vi "FarFiledCamInit.vi"(2 "error in (no error)":errorcluster caption="error in（no error）") -> (0 "error out":errorcluster)   [LabVIEW 2018]
panel:
  out "MinValue":u32
  out "MaxValue":u32
  out "CameraName":string
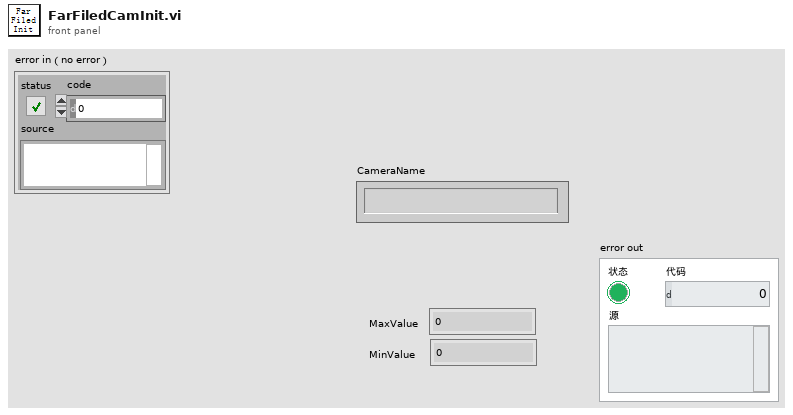
[diagram p1: front panel]
types:
  T1 = typedef "Image Type" = u32
  T2 = typedef "IMAQ Image.ctl" = refnum<image>
  T3 = cluster{"示波器":cluster{"Channel (0:Channel 1)":enum16{"Channel 1", "Channel 2", "Channel 3", "Channel 4"}, "电压范围":dbl, "触发电压":dbl, "时间范围":dbl, " 示波器VISA":refnum<visa-resource-name>, "时间范围 标签":u64, "电压范围 标签":u64, "触发电压 标签":u64, "输入阻抗/Ω":u64}, "光谱仪":cluster{"SpecDataReference":refnum<queue>, "grating center":dbl, "Exposure Time (s)":dbl, "是否进行详细设置":bool, " 开始通信检查":bool, "通信成功？":bool, "波长":dbl}, " 近场相机":cluster{"曝光时间/100us":dbl, "模拟增益":i32, "控制套接字":i32, "IP 地址":string, " 采集套接字":i32, "  版本号":i32, "ImageData":T2, "  增益最大":i32, "  增益最小":i32, " 曝光最大":i32, " 曝光最小":i32, " 帧速":i32, " 同步切换":i32, "  曝光缩放":i32}, " 偏振仪":cluster{"电压范围":u64, "触发电压":u64, "时间范围":u64, "波长范围":enum16{"可见光 400-700nm", "近红外 700-1100nm"}, "可见光偏振测量仪VISA":refnum<visa-resource-name>, "近红外偏振测量仪VISA":refnum<visa-resource-name>}, " 功率计":cluster{"通道":enum16{"Channel 1", "Channel 2"}, "工作波长":u32, "单位":u64, "时间范围":u64, "IP地址":string, "端口":u32}, "能量计":cluster{"通道":enum16{"Channel 1", "Channel 2"}, "工作波长":u32, "单位":u64, "时间范围":u64, "IP地址":string, "端口":u32, "能量计量程":enum16{"200uJ", "20uJ", "2uJ", "200nJ"}}, "电机":cluster{"Channel (0:Channel 1)":enum16{"Channel 1", "Channel 2", "Channel 3", "Channel 4"}, "电压范围":u64, "触发电压":u64, "时间范围":u64}, " 远场相机":cluster{"曝光时间":i32, "模拟增益":i32, "控制套接字":i32, "IP 地址":string, " 采集套接字":i32, "  版本号":i32, "ImageData":T2, "  增益最大":i32, "  增益最小":i32, " 曝光最大":i32, " 曝光最小":i32, " 帧速":i32, " 同步切换":i32, "  曝光缩放":i32, "ImageData B":T2}}
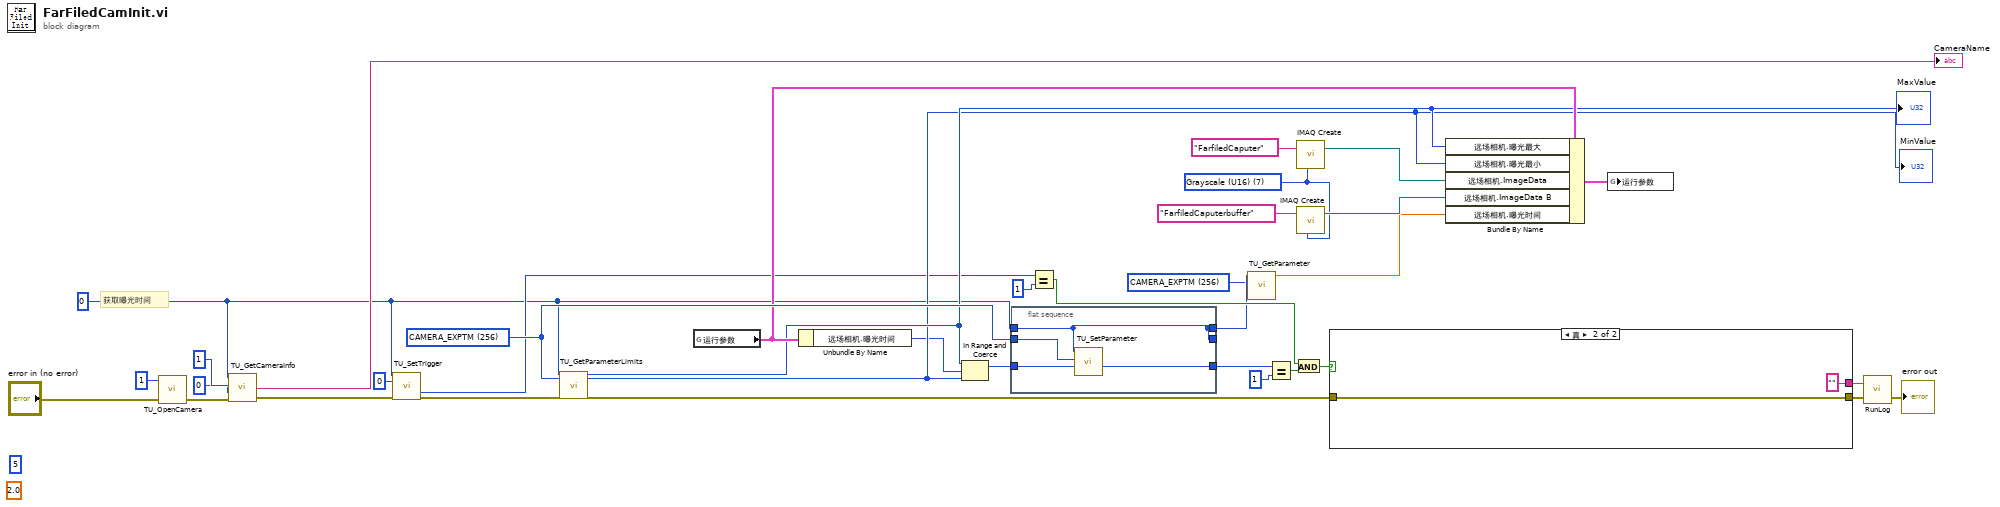
[diagram p0: block diagram]
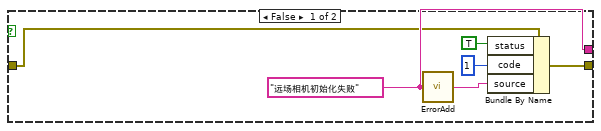
[diagram p2: hidden frame]
diagram:
  w2 = u32 256 items=["CAMERA_EXPTM"=256, "CAMERA_RGAIN"=261, "CAMERA_GGAIN"=266, "CAMERA_BGAIN"=271, "CAMERA_SATURATION"=276, "CAMERA_GAMMA"=281, "CAMERA_CONTRAST"=286] ("Parameter ID")
  w5 = T1 7 items=["Grayscale (U8)", "Grayscale (I16)", "Grayscale (SGL)", "Complex (CSG)", "RGB (U32)", "HSL (U32)", "RGB (U64)", "Grayscale (U16)"] ("Image Type")
  (unwired) 5
  (unwired) 2.0 ("Value in")
  w30 = u32 256 items=["CAMERA_EXPTM"=256, "CAMERA_RGAIN"=261, "CAMERA_GGAIN"=266, "CAMERA_BGAIN"=271, "CAMERA_SATURATION"=276, "CAMERA_GAMMA"=281, "CAMERA_CONTRAST"=286] ("Parameter")
  w11 = u32 0 ("CameraIndex")
  # "获取曝光时间"
  n1 = call "TU_OpenCamera.vi"("error in (no error)"="error in (no error)", "nCamCount"=1) -> ("error out"=w8:errorcluster)  [unwired: 1 in, 2 out]
  n2 = call "TU_GetCameraInfo.vi"("error in (no error)"=w8, "Text Index"=0, "TextID"=1, "CameraIndex"=w11) -> ("error out"=w33:errorcluster, "CameraText"=→"CameraName":string)  [unwired: 1 out]
  n3 = call "TU_SetTrigger.vi"("CameraIndex"=w11, "Capture Mode"=u16 0, "error in (no error)"=w33) -> ("ReturnValue"=w22:u32, "error out"=w31:errorcluster)  [unwired: 11 in]
  n4 = call "TU_GetParameterLimits.vi"("Camera Index"=w11, "Parameter"=w30, "error in (no error)"=w31) -> ("MaxValue"=w28:u32, "MinValue"=w27:u32, "error out"=w6:errorcluster)  [unwired: 11 in, 3 out]
  "MaxValue" <- w28
  "MinValue" <- w27
  n5 = global read "参数.vi" "运行参数"() -> (w29:T3)
  n6 = Unbundle By Name(w29) -> ("远场相机.曝光时间"=w7:i32)
  n7 = In Range and Coerce(upper limit=w28, x=w7, lower limit=w27) -> (coerced(x)=w4:u32)  [unwired: 1 out]
  n8 = flat-sequence {
    tunnel: w30 -> [w40]
    tunnel: [w39] -> w19
    tunnel: w11 -> [w37]
    tunnel: [w37] -> _
    tunnel: w4 -> [w38]
    tunnel: [w37] -> w3
    frame #0 {
      n9 = call "TU_SetParameter.vi"("Value in"=w38, "Parameter"=w40, "Camera Index"=w37) -> ("Return Value"=w39:u32)  [unwired: 4 in]
    }
  }
  n10 = Equal?(x=w22, y=u32 1) -> (x = y?=w18:bool)
  n11 = call "TU_GetParameter.vi"("Parameter ID"=w2, "Camera Index"=w3) -> ("Parameter Value"=w1:dbl)  [unwired: 6 in, 3 out]
  n12 = Equal?(x=w19, y=u32 1) -> (x = y?=w17:bool)
  n13 = And(x=w18, y=w17) -> (x .and. y?=w16:bool)
  n14 = call "IMAQ Create"("Image Name"="FarfiledCaputer", "Image Type"=w5) -> ("New Image"=w14:T2)  [unwired: 3 in, 1 out]
  n15 = call "IMAQ Create"("Image Name"="FarfiledCaputerbuffer", "Image Type"=w5) -> ("New Image"=w12:T2)  [unwired: 3 in, 1 out]
  n16 = case shown="真" w16 {
    tunnel: [w46 ""] -> w25
    tunnel: w6 -> [w43 w48]
    tunnel: [w42 w48] -> w23
    frame False {
      w46 = "远场相机初始化失败" ("source")
      n17 = call "ErrorAdd.vi"("source"=w46) -> ("Errorout Souce"=w44:string)
      n18 = Bundle By Name(cluster=w43, "status"=TRUE, "code"=1, "source"=w44) -> (w42:errorcluster)
    }
    frame True {
    }
  }
  n19 = Bundle By Name(cluster=w29, "远场相机.曝光最大"=w28, "远场相机.曝光最小"=w27, "远场相机.ImageData"=w14, "远场相机.ImageData B"=w12, "远场相机.曝光时间"=w1) -> (w26:T3)
  n20 = global write "参数.vi" "运行参数"(w26) -> ()
  n21 = call "RunLog.vi"("error in"=w23, "Message"=w25) -> ("error out"=→"error out":errorcluster)  [unwired: 1 in]
